vi "Fix Transparency.vi"(10 "Mask":u8[](array[numeric]) format="%.0b", 11 "Pixels In":u32[][](array[numeric]) format="%06x") -> (3 "Pixels Out":u32[][](array[numeric]) format="%06x")   [LabVIEW 2021, in "Utility.lvlib"]
uses:
  Utility.lvlib
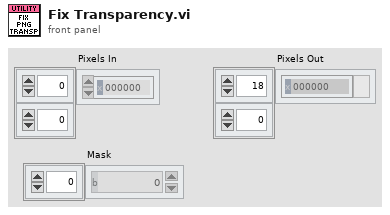
[diagram p1: front panel]
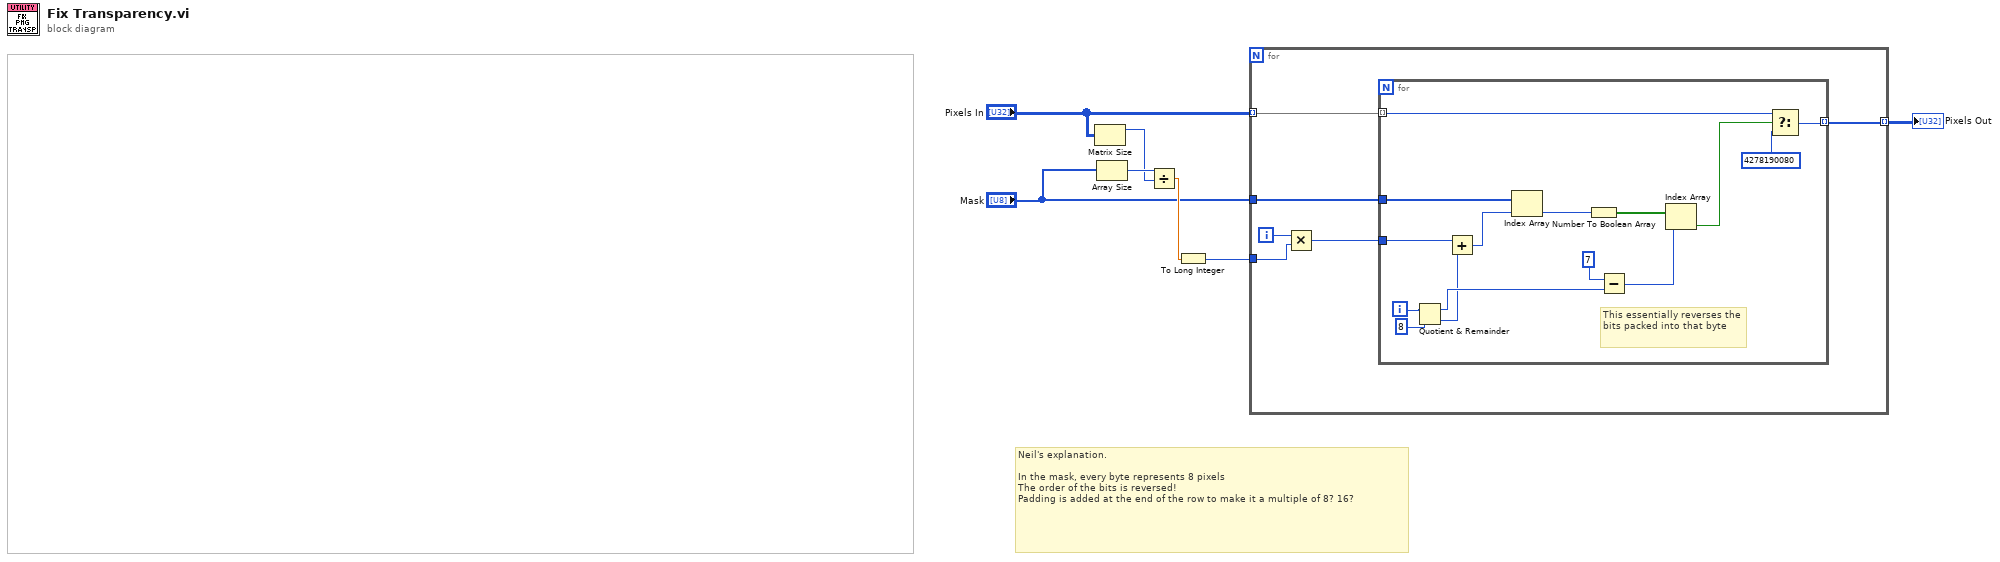
[diagram p0: block diagram]
diagram:
  # "Neil's explanation.\n\nIn the mask, every byte represents 8 pixels\nThe order of the bits is reversed!\nPadding is added at the end of the row to make it a multiple of 8? 16?"
  n1 = Matrix Size(0:"Pixels In") -> (1:w2:i32)  [unwired: 1 out]
  n2 = Array Size(array="Mask") -> (size(s)=w5:i32)
  n3 = Divide(x=w5, y=w2) -> (x/y=w4:dbl)
  n4 = To Long Integer(number=w4) -> (32bit integer=w1:i32)
  n5 = for {
    tunnel: "Pixels In" -> [w13] mode=indexing
    tunnel: [w12] -> w6 mode=indexing
    tunnel: "Mask" -> [w11]
    tunnel: w1 -> [w8]
    i -> [w10]
    n6 = Multiply(x=w10, y=w8) -> (x*y=w9:i32)
    n7 = for {
      tunnel: w13 -> [w27] mode=indexing
      tunnel: [w28] -> w12 mode=indexing
      tunnel: w11 -> [w24]
      tunnel: w9 -> [w15]
      i -> [w20]
      # "This essentially reverses the bits packed into that byte"
      n8 = Quotient & Remainder(x=w20, y=8) -> (x-y*floor(x/y)=w18:i32, floor(x/y)=w17:i32)
      n9 = Add(x=w15, y=w17) -> (x+y=w16:i32)
      n10 = Index Array(array=w24, index=w16) -> (element=w23:u8)
      n11 = Number To Boolean Array(number=w23) -> (Boolean array=w22:bool[])
      n12 = Subtract(x=7, y=w18) -> (x-y=w21:i32)
      n13 = Index Array(array=w22, index=w21) -> (element=w14:bool)
      n14 = Select(t=w27, s=w14, f=u32 4278190080 ("y")) -> (s? t:f=w28:u32)
    }
  }
  "Pixels Out" <- w6
